vi "Or77200_InitDrive.vi"(8 "error In":errorcluster caption="error out", 11 "Port":refnum<visa-resource-name>) -> (0 "sortie d'erreur":errorcluster, 3 "Port Out":refnum<visa-resource-name>)   [LabVIEW 2010]
uses:
  <userlib>/Oriel 77200/OR77200_Init_State.ctl
  <vilib>/Utility/config.llb/Write Key (Double).vi
  <vilib>/Utility/config.llb/NI_LVConfig.lvlib
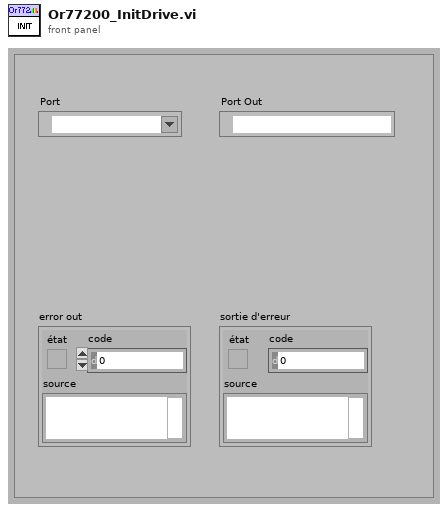
[diagram p1: front panel]
types:
  T1 = typedef "OR77200_Init_State.ctl" = enum16{"Motor Enable", "Clear Position", "Ask Position", "Error"}
  T2 = typedef "NI_LVConfig.lvlib/Config Data RefNum.ctl" = refnum<k1>
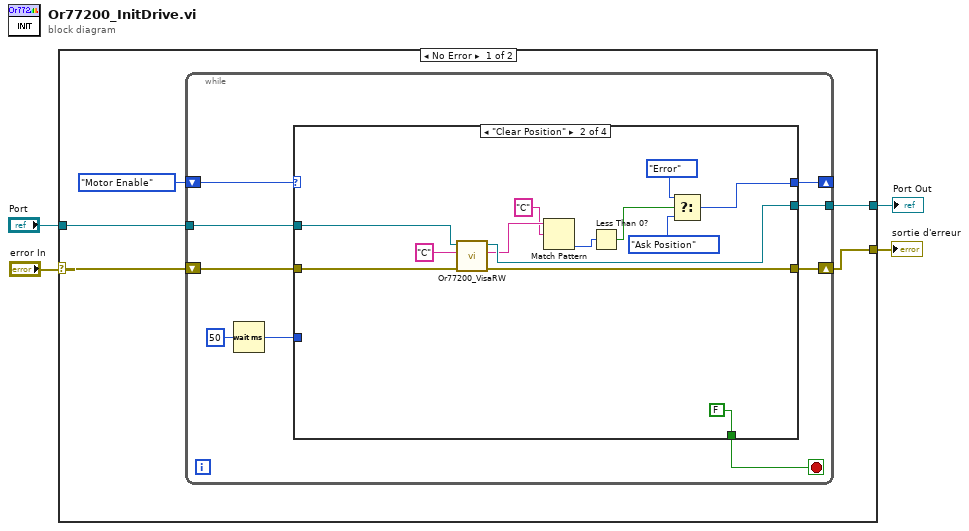
[diagram p0: block diagram]
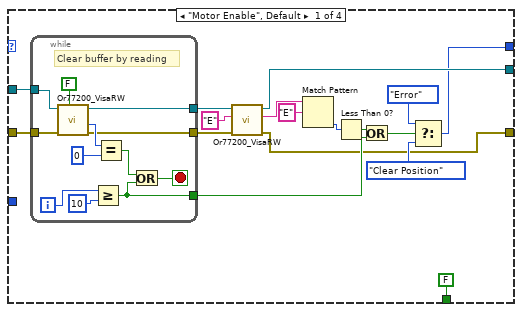
[diagram p2: hidden frame]
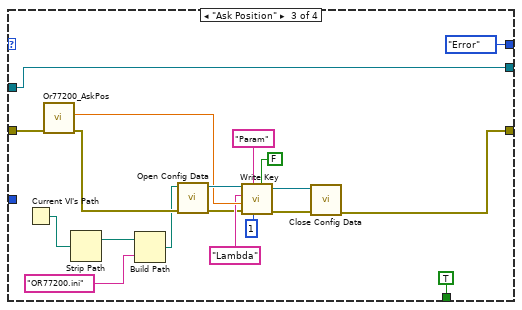
[diagram p3: hidden frame]
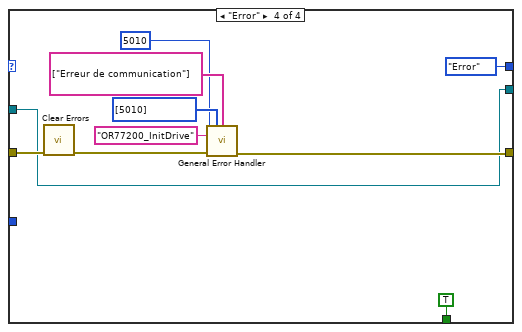
[diagram p4: hidden frame]
diagram:
  n1 = case shown="No Error" "error In" {
    selector: "error In" -> [w7 w90]
    tunnel: "Port" -> [w9 w91]
    tunnel: [w5 w90] -> w3
    tunnel: [w8 w91] -> w2
    frame No Error {
      n2 = while {
        tunnel: w9 -> [w17]
        tunnel: [w16] -> w8
        shift-right: [w13] -> _
        shift-left: OR77200_Init_State."Motor Enable" ("État") -> [w18]
        shift-right: [w14] -> w5
        shift-left: w7 -> [w15]
        stop <- w12 stop-if-true
        n3 = Wait (ms)(milliseconds to wait=u32 50 ("attente (ms)")) -> (millisecond timer value=w11:u32)
        n4 = case shown="\"Clear Position\"" w18 {
          tunnel: w17 -> [w33 w60 w78 w82]
          tunnel: [w35 w53 w78 w82] -> w16
          tunnel: w15 -> [w31 w58 w79 w88]
          tunnel: [w24 w57 w61 w83] -> w14
          tunnel: [w25 w54 OR77200_Init_State."Error" ("État") OR77200_Init_State."Error" ("État")] -> w13
          tunnel: [FALSE FALSE TRUE TRUE] -> w12
          tunnel: w11 -> [_ _ _ _]
          frame "Motor Enable", Default {
            n5 = while {
              tunnel: w33 -> [w39]
              tunnel: [w47] -> w32
              tunnel: w31 -> [w43]
              tunnel: [w37] -> w30
              tunnel: [w36] -> w29
              i -> [w42]
              stop <- w38 stop-if-true
              # "Clear buffer by reading"
              n6 = call <userlib>:"Or77200_VisaRW.vi"("Use LF-Cr"=FALSE, "error in"=w43, "Port"=w39) -> ("error out"=w37:errorcluster, "ByteRead"=w46:u32, "Port Out"=w47:refnum<visa-resource-name>)  [unwired: 5 in, 1 out]
              n7 = Greater Or Equal?(x=w42, y=10) -> (x >= y?=w36:bool)
              n8 = Equal?(x=w46, y=u32 0) -> (x = y?=w40:bool)
              n9 = Or(x=w40, y=w36) -> (x .or. y?=w38:bool)
            }
            n10 = call <userlib>:"Or77200_VisaRW.vi"("error in"=w30, "Commande"="E", "Port"=w32) -> ("error out"=w24:errorcluster, "Response"=w22:string, "Port Out"=w35:refnum<visa-resource-name>)  [unwired: 5 in, 1 out]
            n11 = Match Pattern(string=w22, regular expression="E") -> (offset past match=w20:i32)  [unwired: 1 in, 3 out]
            n12 = Less Than 0?(x=w20) -> (x < 0?=w19:bool)
            n13 = Or(x=w19, y=w29) -> (x .or. y?=w28:bool)
            n14 = Select(t=OR77200_Init_State."Error" ("État"), s=w28, f=OR77200_Init_State."Clear Position" ("État")) -> (s? t:f=w25:T1)
          }
          frame "Clear Position" {
            n15 = call <userlib>:"Or77200_VisaRW.vi"("error in"=w58, "Commande"="C", "Port"=w60) -> ("error out"=w57:errorcluster, "Response"=w50:string, "Port Out"=w53:refnum<visa-resource-name>)  [unwired: 5 in, 1 out]
            n16 = Match Pattern(string=w50, regular expression="C" ("x")) -> (offset past match=w51:i32)  [unwired: 1 in, 3 out]
            n17 = Less Than 0?(x=w51) -> (x < 0?=w48:bool)
            n18 = Select(t=OR77200_Init_State."Error" ("État"), s=w48, f=OR77200_Init_State."Ask Position" ("État")) -> (s? t:f=w54:T1)
          }
          frame "Ask Position" {
            n19 = Current VI's Path() -> (path=w71:path)
            n20 = call <userlib>:"Or77200_AskPos.vi"("error In"=w79) -> ("sortie d'erreur"=w72:errorcluster, "Lambda Out"=w76:dbl)  [unwired: 9 in]
            n21 = Strip Path(path=w71) -> (stripped path=w70:path)  [unwired: 1 out]
            n22 = Build Path(base path=w70, name or relative path="OR77200.ini" ("nom ou chemin relatif")) -> (appended path=w68:path)
            n23 = call <vilib>:"Open Config Data.vi"("error in (no error)"=w72, "configuration file path"=w68) -> ("error out"=w73:errorcluster, "refnum"=w77:T2)  [unwired: 7 in, 1 out]
            n24 = call-poly <vilib>:"Write Key.vi"("use system decimal point (T)"=FALSE, "precision (6)"=i16 1, "section"="Param", "error in (no error)"=w73, "value"=w76, "key"="Lambda", "refnum"=w77) -> ("error out"=w63:errorcluster, "refnum out"=w62:T2)  [unwired: 2 in, 1 out]
            n25 = call <vilib>:"Close Config Data.vi"("error in (no error)"=w63, "refnum"=w62) -> ("error out"=w61:errorcluster)  [unwired: 8 in, 1 out]
          }
          frame "Error" {
            n26 = call <vilib>:"Clear Errors.vi"("error in (no error)"=w88) -> ("error out"=w80:errorcluster)  [unwired: 6 in]
            n27 = call <vilib>:"General Error Handler.vi"("[error code] (0)"=5010, "[user-defined codes]"=i32[] [5010], "[user-defined descriptions]"=string[] ["Erreur de communication"], "[error source] (\" \")"="OR77200_InitDrive" ("[error source] (\" \")"), "error in (no error)"=w80) -> ("error out"=w83:errorcluster)  [unwired: 6 in, 4 out]
          }
        }
      }
    }
    frame Error {
    }
  }
  "sortie d'erreur" <- w3
  "Port Out" <- w2
